vi "string_9_1.vi"() -> ()   [LabVIEW 2026]
panel:
  out "Numeric 2":dbl
  out "s? t:f":string
  out "length 3":i32
  out "length 2":i32
  out "A LEN":dbl
  in  "Numeric":dbl
  in  "B":string
  in  "A":string
  out "concatenated string":string
  in  "Array":string[](array[string])
  in  "String 2":string
  out "length":i32
  in  "String":string
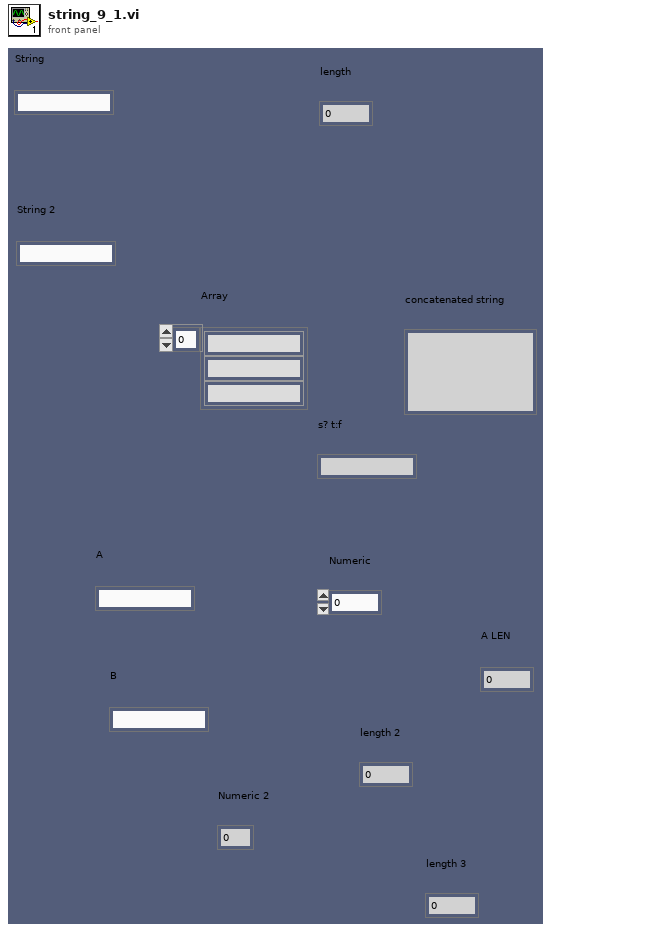
[diagram p1: front panel]
types:
  T1 = cluster{"Array[0]":string, "Array[1]":string, "Array[2]":string, "Array[3]":string, "Array[4]":string, "Array[5]":string, "Array[6]":string, "Array[7]":string, "Array[8]":string}
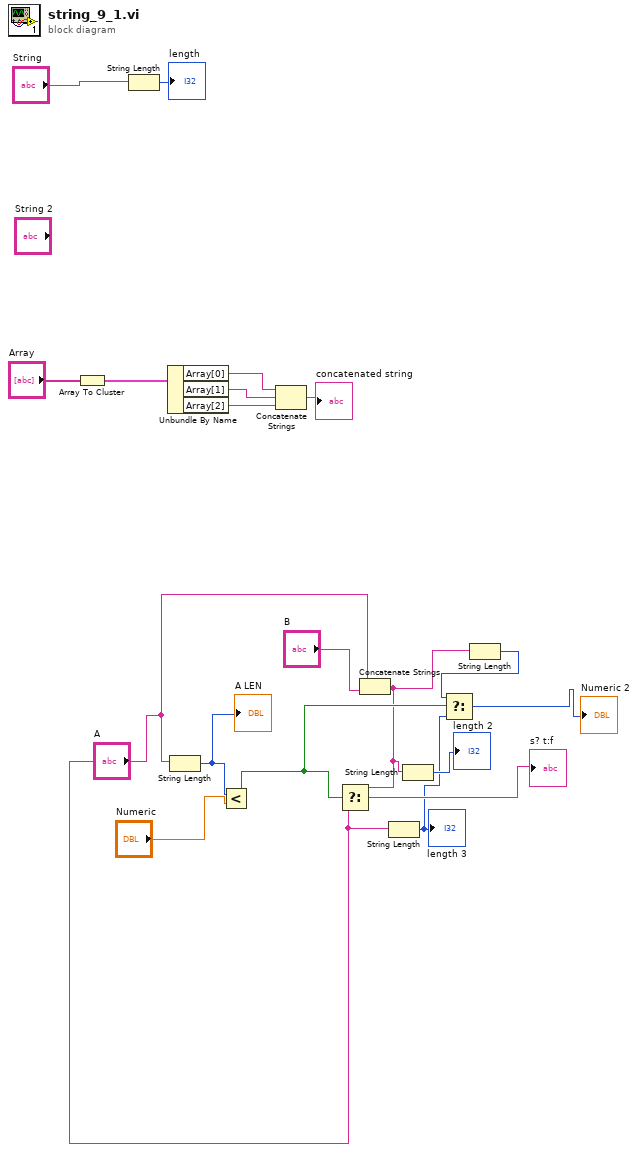
[diagram p0: block diagram]
diagram:
  n1 = Array To Cluster(array="Array") -> (cluster=w16:T1)
  n2 = String Length(string="String") -> (length=→"length":i32)
  n3 = Unbundle By Name(w16) -> ("Array[0]"=w15:string, "Array[1]"=w14:string, "Array[2]"=w13:string)
  n4 = String Length(string="A") -> (length=w11:i32)
  "A LEN" <- w11
  n5 = Less?(x=w11, y="Numeric") -> (x < y?=w5:bool)
  n6 = Concatenate Strings(w15, w14, w13) -> (→"concatenated string":string)
  n7 = Concatenate Strings("A", "B") -> (w3:string)
  n8 = Select(t=w3, s=w5, f="A") -> (s? t:f=→"s? t:f":string)
  n9 = String Length(string="A") -> (length=w1:i32)
  "length 3" <- w1
  n10 = String Length(string=w3) -> (length=→"length 2":i32)
  n11 = String Length(string=w3) -> (length=w2:i32)
  n12 = Select(t=w2, s=w5, f=w1) -> (s? t:f=→"Numeric 2":i32)
